vi "Configure Programmer.vi"(10 "Position":u32, 11 "Program RF in":refnum<class "Program RF.lvclass">) -> (0 "error out":errorcluster, 2 "Programmer out":refnum<class "Segger Flasher ARM.lvclass">)   [LabVIEW 2015, in "Program RF.lvclass"]
doc: "Configures the programmer for RF Programming. Sets up the Segger Serial number, speed, and FW file."
uses:
  Program RF.lvclass
  Classes/Programmer/Segger Flasher ARM/Class/Segger Flasher ARM.lvclass
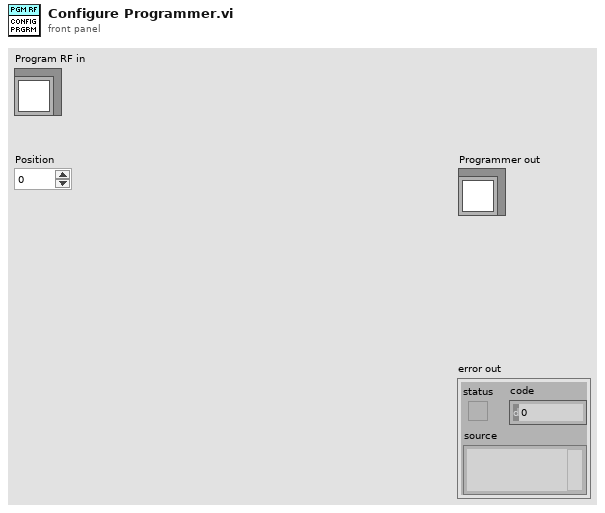
[diagram p1: front panel]
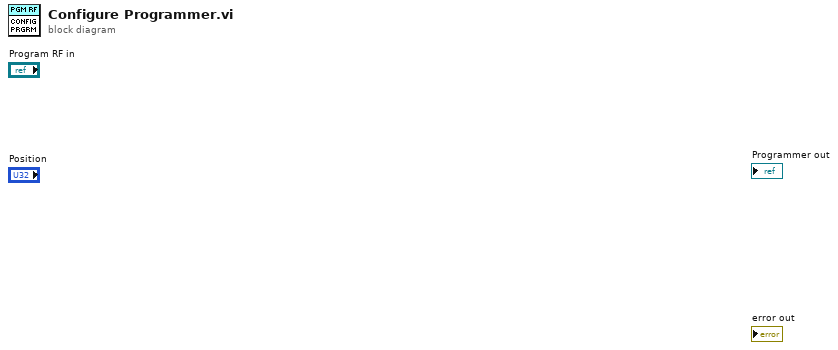
[diagram p0: block diagram]
diagram:
